vi "Generate_Data_Global.vi"() -> ()   [LabVIEW 2023]
panel:
  in  "Generator_Data":dbl
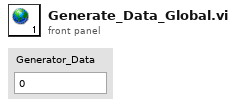
[diagram p1: front panel]
diagram:
